vi "GetSampleInfo.vi"(0 "TCP网络连接输入":refnum<k5>, 11 "错误输入（无错误）":errorcluster) -> (6 "TCP网络连接输入 2":refnum<k5>, 8 "值":string[][](array[string]), 10 "错误输出 2":errorcluster caption="错误输出", 15 "错误输出":errorcluster)   [LabVIEW 2014]
panel:
  out "连接的字符串":string
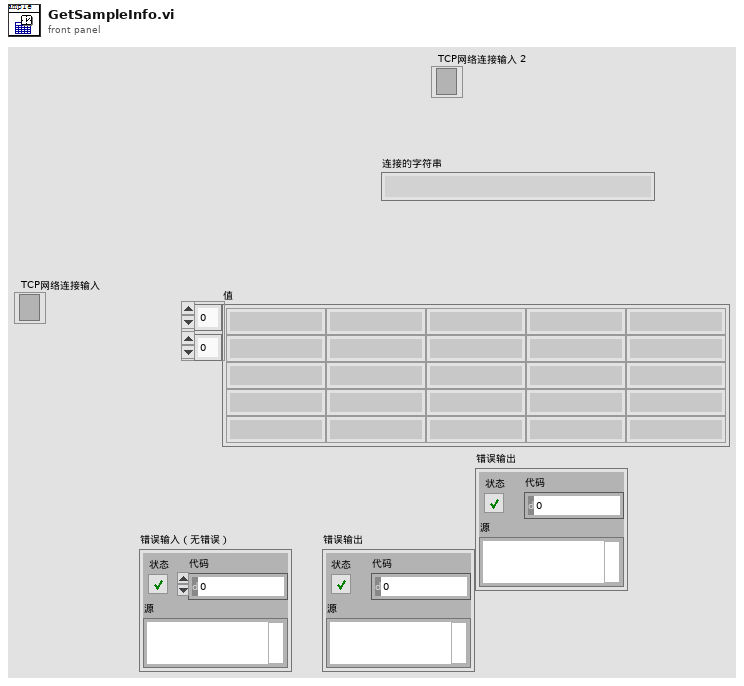
[diagram p1: front panel]
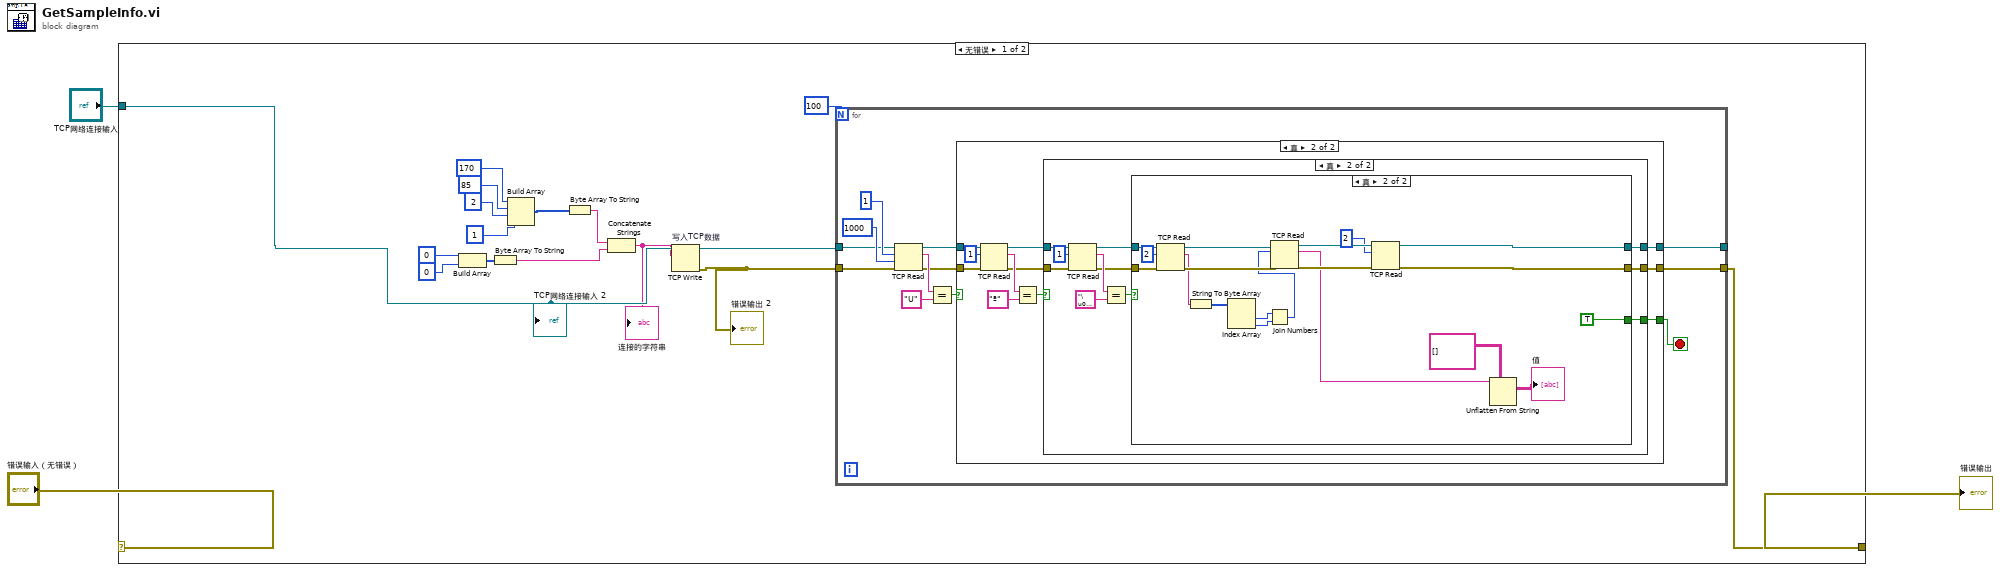
[diagram p0: block diagram]
diagram:
  n1 = case shown="无错误" "错误输入（无错误）" {
    selector: "错误输入（无错误）" -> [_ w79]
    tunnel: [w15 w79] -> w3
    tunnel: "TCP网络连接输入" -> [w16 _]
    frame No Error {
      n2 = Build Array(u8 0, u8 0) -> (w8:u8[])
      n3 = Byte Array To String(unsigned byte array=w8) -> (string=w4:string)
      n4 = Build Array(u8 170, u8 85, u8 2, u8 1) -> (w11:u8[])
      n5 = Byte Array To String(unsigned byte array=w11) -> (string=w7:string)
      n6 = Concatenate Strings(w7, w4) -> (w6:string)
      "连接的字符串" <- w6
      n7 = TCP Write "写入TCP数据"(connection ID=w16, data in=w6) -> (connection ID out=w19:refnum<k5>, error out=w18:errorcluster)  [unwired: 2 in, 1 out]
      "错误输出 2" <- w18
      n8 = for "For循环" {
        N: 100 -> [_]
        tunnel: w19 -> [w24]
        tunnel: [w21] -> _
        tunnel: w18 -> [w23]
        tunnel: [w20] -> w15
        stop <- w22 stop-if-true
        n9 = TCP Read(connection ID=w24, bytes to read=1 ("读取的字节"), error in (no error)=w23, 9:1000 ("超时毫秒(25000)")) -> (connection ID out=w27:refnum<k5>, data out=w29:string, error out=w26:errorcluster)  [unwired: 1 in]
        n10 = Equal?(x=w29, y="U") -> (x = y?=w28:bool)
        n11 = case shown="真" w28 {
          tunnel: w27 -> [w33 w41]
          tunnel: w26 -> [w32 w40]
          tunnel: [w33 w36] -> w21
          tunnel: [w32 w35] -> w20
          tunnel: [_ w34] -> w22
          frame False {
          }
          frame True {
            n12 = TCP Read(connection ID=w41, bytes to read=1 ("读取的字节"), error in (no error)=w40) -> (connection ID out=w38:refnum<k5>, data out=w42:string, error out=w37:errorcluster)  [unwired: 2 in]
            n13 = Equal?(x=w42, y="ª") -> (x = y?=w39:bool)
            n14 = case shown="真" w39 {
              tunnel: w38 -> [w46 w54]
              tunnel: w37 -> [w45 w53]
              tunnel: [w46 w49] -> w36
              tunnel: [w45 w48] -> w35
              tunnel: [_ w47] -> w34
              frame False {
              }
              frame True {
                n15 = TCP Read(connection ID=w54, bytes to read=1 ("读取的字节"), error in (no error)=w53) -> (connection ID out=w52:refnum<k5>, data out=w55:string, error out=w51:errorcluster)  [unwired: 2 in]
                n16 = Equal?(x=w55, y="\u0002") -> (x = y?=w50:bool)
                n17 = case shown="真" w50 {
                  tunnel: w52 -> [w59 w77]
                  tunnel: w51 -> [w58 w76]
                  tunnel: [w59 w69] -> w49
                  tunnel: [w58 w70] -> w48
                  tunnel: [_ TRUE] -> w47
                  frame False {
                  }
                  frame True {
                    n18 = TCP Read(connection ID=w77, bytes to read=2 ("读取的字节"), error in (no error)=w76) -> (connection ID out=w75:refnum<k5>, data out=w64:string, error out=w74:errorcluster)  [unwired: 2 in]
                    n19 = String To Byte Array(string=w64) -> (unsigned byte array=w63:u8[])
                    n20 = Index Array(array=w63) -> (element #1=w62:u8, element #2=w61:u8)  [unwired: 2 in]
                    n21 = Join Numbers(hi=w62, lo=w61) -> ((hi.lo)=w60:u16)
                    n22 = TCP Read(connection ID=w75, bytes to read=w60, error in (no error)=w74) -> (connection ID out=w72:refnum<k5>, data out=w67:string, error out=w71:errorcluster)  [unwired: 2 in]
                    n23 = TCP Read(connection ID=w72, bytes to read=2 ("读取的字节"), error in (no error)=w71) -> (connection ID out=w69:refnum<k5>, error out=w70:errorcluster)  [unwired: 2 in, 1 out]
                    n24 = Unflatten From String(type=string[][] [], binary string=w67) -> (value=→"值":string[][])  [unwired: 3 in, 2 out]
                  }
                }
              }
            }
          }
        }
      }
      "TCP网络连接输入 2" <- w16
    }
    frame Error {
    }
  }
  "错误输出" <- w3
